vi "Manual View.vi"() -> ()   [LabVIEW 2016, in "HPMT_Views.lvlib"]
uses:
  HPMT_Views.lvlib
  User Events/User Events.lvclass
  Commands/Command Factory/Command Factory.lvclass
  User Events/User Events.lvclass/User Events.ctl
  Typedefs/StateTypes.ctl
  Commands/Move Steps Command/Move Steps Command.lvclass
  Commands/Stop Constant Query Command/Stop Constant Query Command.lvclass
  Commands/Constant Query Command/Constant Query Command.lvclass
  Commands/Search For Zero Command/Search For Zero.lvclass
  Commands/Complete Manual Command/Complete Manual Command.lvclass
  Globals.vi
  Typedefs/HPMT_Typedefs.lvlib
panel:
  in  "Search For Zero":bool
  in  "Constant Query":bool
  in  "Number Of Steps":i32
  in  "Complete Manual":bool
  in  "User Events in":refnum<class "User Events.lvclass">
  in  "Move Steps":bool
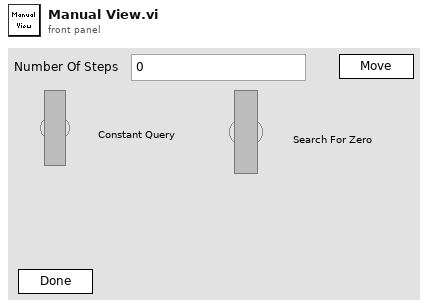
[diagram p1: front panel]
types:
  T1 = typedef "HPMT_Typedefs.lvlib/Publish Data Events.ctl" = cluster{"State":refnum<user-event>, "ErrorCode":refnum<user-event>, "Scan Progress":refnum<user-event>, "All Test Status":refnum<user-event>, "ActuatorData":refnum<user-event>, "Test Settings":refnum<user-event>, "Stop Constant Query":refnum<user-event>}
  T2 = typedef "HPMT_Typedefs.lvlib/Subscribe Data Events.ctl" = cluster{"Command":refnum<user-event>}
  T3 = typedef "HPMT_Typedefs.lvlib/StateTypes.ctl" = enum16{"Offline State", "Fault State", "Standby State", "Disabled State", "Enabled State", "Wait For User Input State", "Test Actuator State", "Manual State"}
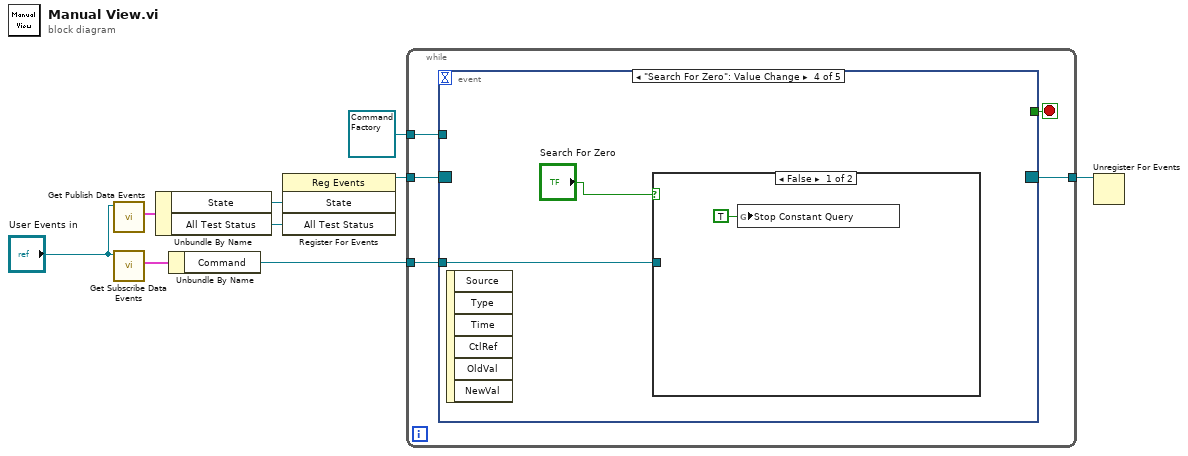
[diagram p0: block diagram]
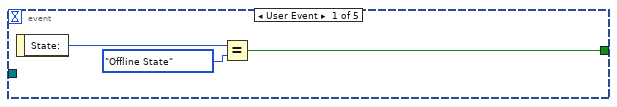
[diagram p2: hidden frame]
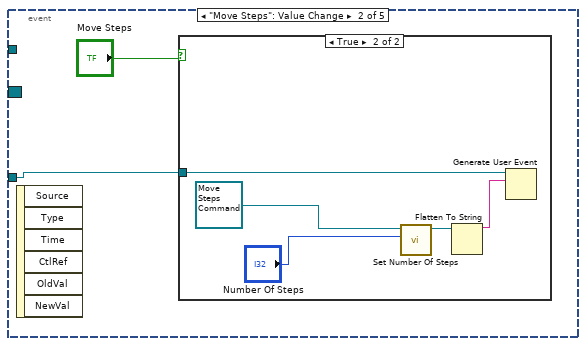
[diagram p3: hidden frame]
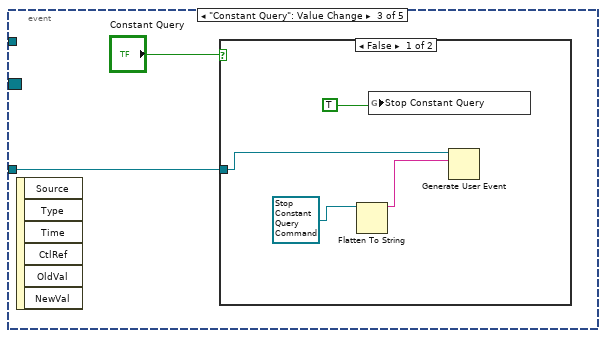
[diagram p5: hidden frame]
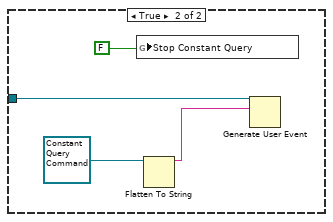
[diagram p6: hidden frame]
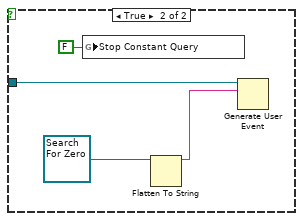
[diagram p7: hidden frame]
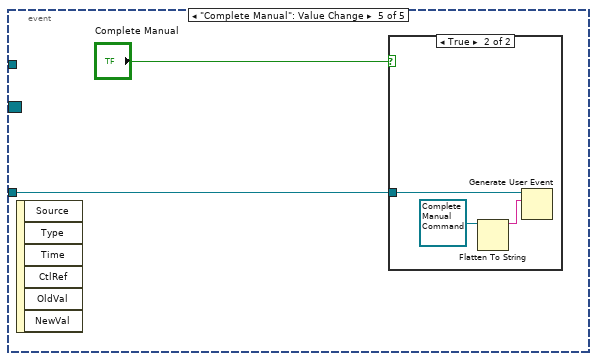
[diagram p8: hidden frame]
diagram:
  n1 = call "Get Publish Data Events.vi"("UserEvents in"="User Events in") -> ("Publish Data Events"=w7:T1)  [unwired: 9 in, 1 out]
  n2 = call "Get Subscribe Data Events.vi"("UserEvents in"="User Events in") -> ("Subscribe Data Events"=w8:T2)  [unwired: 9 in, 1 out]
  n3 = Unbundle By Name(w7) -> ("State"=w6:refnum<user-event>, "All Test Status"=w5:refnum<user-event>)
  n4 = Unbundle By Name(w8) -> ("Command"=w3:refnum<user-event>)
  n5 = register-events(w6, w5) -> (reference out=w2:refnum<event-registration>)  [unwired: 2 in, 1 out]
  n6 = while {
    tunnel: refnum<class "Command Factory.lvclass"> refnum ("Command Factory.lvclass") -> [w14]
    tunnel: w3 -> [w13]
    tunnel: w2 -> [w12]
    tunnel: [w10] -> w1
    stop <- w11 stop-if-true
    n7 = event shown="[3] \"Search For Zero\": Value Change" {
      selector: w12 -> [_ _ _ _ _]
      dyn-events: [_ _ _ _ _] -> w10
      timeout: _ -> [_ _ _ _ _]
      tunnel: w14 -> [_ _ _ _ _]
      tunnel: w13 -> [_ w18 w25 w35 w42]
      tunnel: [w15 _ _ _ _] -> w11
      event User Event {
        n8 = event-data() -> ("State:"=w17:T3)  [unwired: 1 in]
        n9 = Equal?(x=w17, y=StateTypes."Offline State") -> (x = y?=w15:bool)
      }
      event "Move Steps": Value Change {
        n10 = event-data() -> ()  [unwired: 1 in, 6 out]
        n11 = case shown="True" "Move Steps" {
          tunnel: w18 -> [_ w24]
          frame False {
          }
          frame True {
            n12 = call "Set Number Of Steps.vi"("Number Of Steps"="Number Of Steps", "Move Steps Command in"=refnum<class "Move Steps Command.lvclass"> refnum ("Move Steps Command.lvclass")) -> ("Move Steps Command out"=w21:refnum<class "Move Steps Command.lvclass">)  [unwired: 9 in]
            n13 = Flatten To String(anything=w21) -> (data string=w23:string)  [unwired: 3 in, 2 out]
            n14 = Generate User Event(user event=w24, event data cluster=w23) -> ()  [unwired: 2 in, 2 out]
          }
        }
      }
      event "Constant Query": Value Change {
        n15 = event-data() -> ()  [unwired: 1 in, 6 out]
        n16 = case shown="False" "Constant Query" {
          tunnel: w25 -> [w28 w34]
          frame False {
            n17 = Flatten To String(anything=refnum<class "Stop Constant Query Command.lvclass"> refnum ("Stop Constant Query Command.lvclass")) -> (data string=w29:string)  [unwired: 3 in, 2 out]
            n18 = global write "Globals.vi" "Stop Constant Query"(TRUE) -> ()
            n19 = Generate User Event(user event=w28, event data cluster=w29) -> ()  [unwired: 2 in, 2 out]
          }
          frame True {
            n20 = global write "Globals.vi" "Stop Constant Query"(FALSE) -> ()
            n21 = Flatten To String(anything=refnum<class "Constant Query Command.lvclass"> refnum ("Constant Query Command.lvclass")) -> (data string=w32:string)  [unwired: 3 in, 2 out]
            n22 = Generate User Event(user event=w34, event data cluster=w32) -> ()  [unwired: 2 in, 2 out]
          }
        }
      }
      event "Search For Zero": Value Change {
        n23 = event-data() -> ()  [unwired: 1 in, 6 out]
        n24 = case shown="False" "Search For Zero" {
          tunnel: w35 -> [_ w40]
          frame False {
            n25 = global write "Globals.vi" "Stop Constant Query"(TRUE ("Stop Constant Query")) -> ()
          }
          frame True {
            n26 = global write "Globals.vi" "Stop Constant Query"(FALSE ("Stop Constant Query")) -> ()
            n27 = Flatten To String(anything=refnum<class "Search For Zero.lvclass"> refnum ("Search For Zero.lvclass")) -> (data string=w38:string)  [unwired: 3 in, 2 out]
            n28 = Generate User Event(user event=w40, event data cluster=w38) -> ()  [unwired: 2 in, 2 out]
          }
        }
      }
      event "Complete Manual": Value Change {
        n29 = event-data() -> ()  [unwired: 1 in, 6 out]
        n30 = case shown="True" "Complete Manual" {
          tunnel: w42 -> [_ w44]
          frame False {
          }
          frame True {
            n31 = Flatten To String(anything=refnum<class "Complete Manual Command.lvclass"> refnum ("Complete Manual Command.lvclass")) -> (data string=w45:string)  [unwired: 3 in, 2 out]
            n32 = Generate User Event(user event=w44, event data cluster=w45) -> ()  [unwired: 2 in, 2 out]
          }
        }
      }
    }
  }
  n33 = Unregister For Events(event registration refnum=w1) -> ()  [unwired: 1 in, 1 out]
